vi "New_camera_testcode.vi"() -> ()   [LabVIEW 2024]
uses:
  <vilib>/vision/driver/IMAQdx.llb/IMAQdx Camera Control Mode.ctl
  Camera_ID.ctl
  <vilib>/vision/driver/IMAQdx.llb/IMAQdx Acquisition Mode.ctl
  <vilib>/vision/driver/IMAQdx.llb/IMAQdx Buffer Number Mode.ctl
  <vilib>/vision/driver/NI_Vision_Acquisition_Software.lvlib
panel:
  out "error out 2":errorcluster
  out "error out":errorcluster
  out "Cal2":path
  out "Cal1":path
  out "error out 4":errorcluster
  out "error out 3":errorcluster
  out "Image 4":T1(plugin-control)
  out "Image 3":T1(plugin-control)
  out "CAM1":string
  out "CAM2":string
  in  "Exposure time":dbl=2000.0
  in  "stop":bool
  in  "CAM_ID2":i32=23466442
  in  "CAM_ID1":i32=30088089
  in  "Frames pr. sek.":dbl=15.0
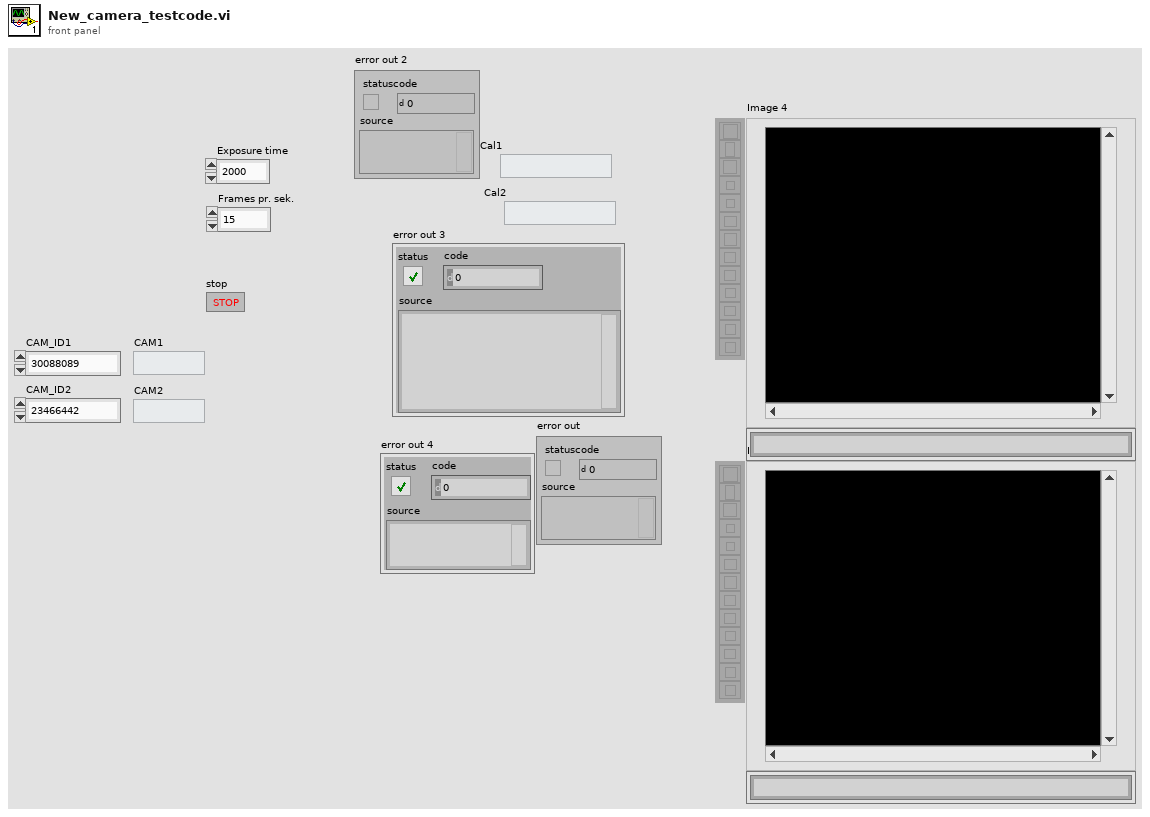
[diagram p1: front panel]
types:
  T1 = typedef "IMAQ Image.ctl" = refnum<image>
  T2 = typedef "NI_Vision_Acquisition_Software.lvlib/IMAQdx Acquisition Mode.ctl" = enum32{"One Shot", "Continuous"}
  T3 = typedef "Camera_ID.ctl" = enum16{"Camera 1", "Camera 2"}
  T4 = typedef "NI_Vision_Acquisition_Software.lvlib/IMAQdx Camera Control Mode.ctl" = enum32{"Controller", "Listener"}
  T5 = typedef "IMAQdx.ctl" = refnum<k21>
  T6 = typedef "NI_Vision_Acquisition_Software.lvlib/IMAQdx Buffer Number Mode.ctl" = enum32{"Next", "Last", "Buffer Number", "Every", "Last New"}
  T7 = typedef "Image Type" = u32
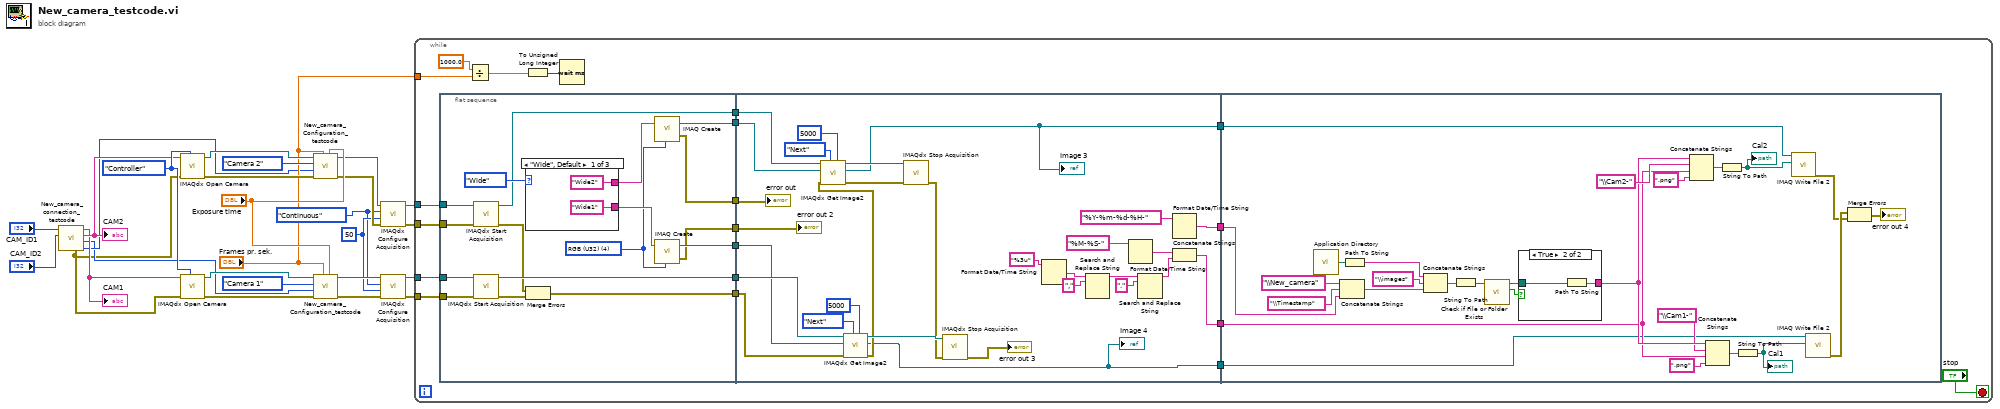
[diagram p0: block diagram]
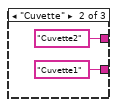
[diagram p2: hidden frame]
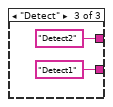
[diagram p3: hidden frame]
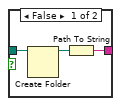
[diagram p4: hidden frame]
diagram:
  w1 = IMAQdx_Acquisition_Mode."Continuous" ("Continuous?")
  w2 = u32 50 ("Number of Buffers")
  w26 = IMAQdx_Camera_Control_Mode."Controller" ("Camera Control Mode")
  n1 = call "New_camera_connection_testcode.vi"("CAM_ID2"="CAM_ID2", "CAM_ID1"="CAM_ID1") -> ("CAM2 Model"=w13:enum16{"a2A5328-15ucBAS", "acA1920-155uc"}, "CAM1 Model"=w12:enum16{"a2A5328-15ucBAS", "acA1920-155uc"}, "CAM2"=w25:string, "CAM1"=w24:string, "error out"=w11:errorcluster)  [unwired: 5 in]
  "CAM2" <- w25
  "CAM1" <- w24
  n2 = call <vilib>:"IMAQdx Open Camera.vi"("Camera Control Mode"=w26, "error in"=w11, "Session In"=w25) -> ("error out"=w16:errorcluster, "Session Out"=w19:T5)  [unwired: 7 in]
  n3 = call <vilib>:"IMAQdx Open Camera.vi"("Camera Control Mode"=w26, "error in"=w11, "Session In"=w24) -> ("error out"=w17:errorcluster, "Session Out"=w18:T5)  [unwired: 7 in]
  n4 = call "New_camera_Configuration_testcode.vi"("Exposure time"="Exposure time", "Framerate"="Frames pr. sek.", "error in (no error)"=w16, "CAM Model"=w13, "Camera"=Camera_ID."Camera 2", "Refnum in"=w19) -> ("error out 2"=w7:errorcluster, "Refnum out 2"=w10:T5)  [unwired: 4 in]
  n5 = call "New_camera_Configuration_testcode.vi"("Exposure time"="Exposure time", "Framerate"="Frames pr. sek.", "error in (no error)"=w17, "CAM Model"=w12, "Camera"=Camera_ID."Camera 1", "Refnum in"=w18) -> ("error out 2"=w4:errorcluster, "Refnum out 2"=w5:T5)  [unwired: 4 in]
  n6 = call <vilib>:"IMAQdx Configure Acquisition.vi"("error in"=w7, "Number of Buffers"=w2, "Continuous?"=w1, "Session In"=w10) -> ("error out"=w8:errorcluster, "Session Out"=w9:T5)  [unwired: 6 in]
  n7 = call <vilib>:"IMAQdx Configure Acquisition.vi"("error in"=w4, "Number of Buffers"=w2, "Continuous?"=w1, "Session In"=w5) -> ("error out"=w3:errorcluster, "Session Out"=w6:T5)  [unwired: 6 in]
  n8 = while {
    tunnel: "Frames pr. sek." -> [w33]
    tunnel: w8 -> [w32]
    tunnel: w9 -> [w31]
    tunnel: w3 -> [w30]
    tunnel: w6 -> [w29]
    stop <- "stop" stop-if-true
    n9 = flat-sequence {
      tunnel: [w59] -> w42
      tunnel: [w58] -> w41
      tunnel: [w57] -> w40
      tunnel: [w56] -> w39
      tunnel: [w53] -> w38
      tunnel: w32 -> [w51]
      tunnel: w31 -> [w52]
      tunnel: w30 -> [w49]
      tunnel: w29 -> [w50]
      tunnel: [w48] -> w28
      tunnel: [w47] -> w27
      tunnel: w42 -> [w91]
      tunnel: w41 -> [w90]
      tunnel: w40 -> [w73]
      tunnel: w39 -> [w89]
      tunnel: w38 -> [w88]
      tunnel: [w78] -> w37
      tunnel: [w76] -> w36
      tunnel: [w75] -> w35
      tunnel: [w72] -> w34
      tunnel: w28 -> [w71]
      tunnel: w27 -> [w70]
      tunnel: w37 -> [w107]
      tunnel: w36 -> [w112]
      tunnel: w35 -> [w100]
      tunnel: w34 -> [w102]
      frame #0 {
        w60 = T7 4 items=["Grayscale (U8)", "Grayscale (I16)", "Grayscale (SGL)", "Complex (CSG)", "RGB (U32)", "HSL (U32)", "RGB (U64)", "Grayscale (U16)"] ("Image Type")
        n10 = call <vilib>:"IMAQdx Start Acquisition.vi"("error in"=w51, "Session In"=w52) -> ("error out"=w54:errorcluster, "Session Out"=w58:T5)  [unwired: 8 in]
        n11 = call <vilib>:"IMAQdx Start Acquisition.vi"("error in"=w49, "Session In"=w50) -> ("error out"=w55:errorcluster, "Session Out"=w59:T5)  [unwired: 8 in]
        n12 = case shown="\"Wide\", Default" enum16{"Wide", "Cuvette", "Detect"}."Wide" {
          tunnel: ["Wide1" "Cuvette1" "Detect1"] -> w62
          tunnel: ["Wide2" "Cuvette2" "Detect2"] -> w61
          frame "Wide", Default {
          }
          frame "Cuvette" {
          }
          frame "Detect" {
          }
        }
        n13 = Merge Errors(w54, w55) -> (w53:errorcluster)
        n14 = call "IMAQ Create"("Image Name"=w61, "Image Type"=w60) -> ("New Image"=w56:T1, "error out"=w48:errorcluster)  [unwired: 3 in]
        n15 = call "IMAQ Create"("Image Name"=w62, "Image Type"=w60) -> ("New Image"=w57:T1, "error out"=w47:errorcluster)  [unwired: 3 in]
      }
      frame #1 {
        n16 = call <vilib>:"IMAQdx Get Image2.vi"("Timeout (ms)"=5000, "Buffer Number Mode (Next)"=IMAQdx_Buffer_Number_Mode."Next", "error in"=w88, "Image In"=w73, "Session In"=w91) -> ("error out"=w74:errorcluster, "Image Out"=w72:T1, "Session Out"=w98:T5)  [unwired: 3 in, 1 out]
        "Image 4" <- w72
        n17 = call <vilib>:"IMAQdx Get Image2.vi"("Timeout (ms)"=5000, "Buffer Number Mode (Next)"=IMAQdx_Buffer_Number_Mode."Next", "error in"=w74, "Image In"=w89, "Session In"=w90) -> ("error out"=w93:errorcluster, "Image Out"=w75:T1, "Session Out"=w99:T5)  [unwired: 3 in, 1 out]
        "Image 3" <- w75
        n18 = call <vilib>:"IMAQdx Stop Acquisition.vi"("error in"=w93, "Session In"=w99) -> ("error out"=w92:errorcluster)  [unwired: 8 in, 1 out]
        n19 = call <vilib>:"IMAQdx Stop Acquisition.vi"("error in"=w92, "Session In"=w98) -> ("error out"=→"error out 3":errorcluster)  [unwired: 8 in, 1 out]
        n20 = Format Date/Time String(time format string (%c)="%3u") -> (date/time string=w86:string)  [unwired: 2 in]
        n21 = Search and Replace String(input string=w86, search string=",") -> (result string=w80:string)  [unwired: 6 in, 3 out]
        n22 = Format Date/Time String(time format string (%c)="%M-%S-") -> (date/time string=w85:string)  [unwired: 2 in]
        n23 = Search and Replace String(input string=w80, search string=".") -> (result string=w79:string)  [unwired: 6 in, 3 out]
        n24 = Format Date/Time String(time format string (%c)="%Y-%m-%d-%H-") -> (date/time string=w76:string)  [unwired: 2 in]
        n25 = Concatenate Strings(w85, w79) -> (w78:string)
        "error out" <- w71
        "error out 2" <- w70
      }
      frame #2 {
        n26 = call <vilib>:"Application Directory.vi"() -> ("Application Directory"=w122:path)
        n27 = Concatenate Strings("\\New_camera" ("string"), "\\Timestamp" ("string"), w112) -> (w101:string)
        n28 = Path To String(path=w122) -> (string=w117:string)
        n29 = Concatenate Strings(w117, "\\images" ("string"), w101) -> (w115:string)
        n30 = String To Path(string=w115) -> (path=w123:path)
        n31 = call <vilib>:"Check if File or Folder Exists.vi"("path"=w123) -> ("file or folder exists?"=w125:bool, "dup path"=w124:path)  [unwired: 8 in, 1 out]
        n32 = case shown="True" w125 {
          tunnel: w124 -> [w128 w130]
          tunnel: [w126 w129] -> w109
          frame False {
            n33 = Create Folder(path (use dialog)=w128) -> (created path=w127:path)  [unwired: 2 in, 2 out]
            n34 = Path To String(path=w127) -> (string=w126:string)
          }
          frame True {
            n35 = Path To String(path=w130) -> (string=w129:string)
          }
        }
        n36 = Concatenate Strings(w109, "\\Cam2-" ("string"), w107, ".png" ("string")) -> (w120:string)
        n37 = Concatenate Strings(w109, "\\Cam1-" ("string"), w107, ".png" ("string")) -> (w106:string)
        n38 = String To Path(string=w120) -> (path=w118:path)
        "Cal2" <- w118
        n39 = String To Path(string=w106) -> (path=w119:path)
        "Cal1" <- w119
        n40 = call-poly "IMAQ Write File 2"("File Path"=w118, "Image"=w100) -> ("error out"=w104:errorcluster)  [unwired: 8 in, 1 out]
        n41 = call-poly "IMAQ Write File 2"("File Path"=w119, "Image"=w102) -> ("error out"=w105:errorcluster)  [unwired: 8 in, 1 out]
        n42 = Merge Errors(w105, w104) -> (→"error out 4":errorcluster)
      }
    }
    n43 = Divide(x=1000.0, y=w33) -> (x/y=w45:dbl)
    n44 = To Unsigned Long Integer(number=w45) -> (unsigned 32bit integer=w44:u32)
    n45 = Wait (ms)(milliseconds to wait=w44) -> ()  [unwired: 1 out]
  }
